vi "Query Voltage Range.vi"(8 "error in (no error)":errorcluster, 11 "VISA resource name":refnum<visa-resource-name>) -> (0 "error out":errorcluster, 1 "Maximum value":u16, 2 "Minimum value":u16, 3 "VISA resource name out":refnum<visa-resource-name>)   [LabVIEW 2013, in "IT6900.lvlib"]
doc: "Provides the range of values for query voltage. Output minimum and maximum value."
uses:
  IT6900.lvlib
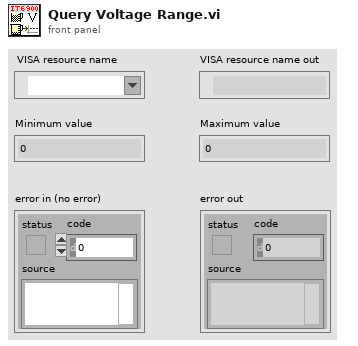
[diagram p1: front panel]
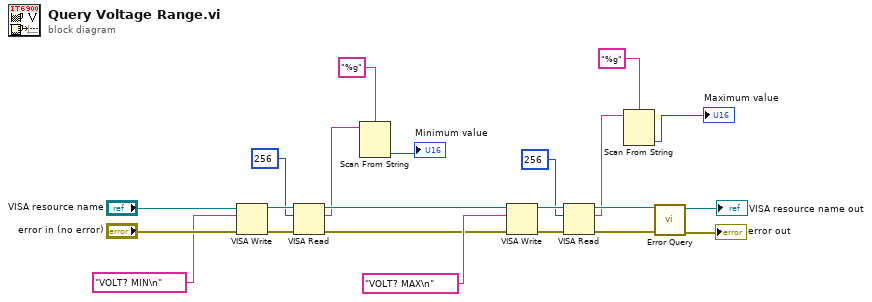
[diagram p0: block diagram]
diagram:
  n1 = VISA Write(VISA resource name="VISA resource name", write buffer="VOLT? MIN\n", error in (no error)="error in (no error)") -> (VISA resource name out=w18:refnum<visa-resource-name>, error out=w19:errorcluster)  [unwired: 1 out]
  n2 = VISA Read(VISA resource name=w18, byte count=256, error in (no error)=w19) -> (VISA resource name out=w12:refnum<visa-resource-name>, read buffer=w6:string, error out=w11:errorcluster)  [unwired: 1 out]
  n3 = Scan From String(format string="%g", input string=w6) -> (output 1=→"Minimum value":u16)  [unwired: 3 in, 3 out]
  n4 = VISA Write(VISA resource name=w12, write buffer="VOLT? MAX\n", error in (no error)=w11) -> (VISA resource name out=w15:refnum<visa-resource-name>, error out=w16:errorcluster)  [unwired: 1 out]
  n5 = VISA Read(VISA resource name=w15, byte count=256, error in (no error)=w16) -> (VISA resource name out=w9:refnum<visa-resource-name>, read buffer=w3:string, error out=w10:errorcluster)  [unwired: 1 out]
  n6 = Scan From String(format string="%g", input string=w3) -> (output 1=→"Maximum value":u16)  [unwired: 3 in, 3 out]
  n7 = call "Error Query.vi"("error in (no error)"=w10, "VISA resource name"=w9) -> ("error out"=→"error out":errorcluster, "VISA resource name out"=→"VISA resource name out":refnum<visa-resource-name>)  [unwired: 6 in, 2 out]
